vi "Vision Processing.vi"(4 "error in (no error)":errorcluster) -> ()   [LabVIEW 2013]
doc: "This VI runs in parallel to other tasks. It gets images from the camera, processes them for color or shape and use that information to affect robot behavior."
uses:
  Robot Global Data.vi
  <vilib>/Rock Robotics/WPI/Solenoid/Deprecated/WPI_SolenoidSetBool.vi
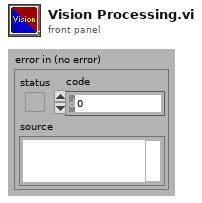
[diagram p1: front panel]
types:
  T1 = typedef "Image Type" = u32
  T2 = typedef "WPI_CameraDevRef.ctl" = cluster{"Camera Address":string, "CameraStatus":errorcluster, "Acquire Image Notifier":refnum<notifier>}
  T3 = typedef "IMAQ Image.ctl" = refnum<image>
  T4 = typedef "WPI_SolenoidDevRef.ctl" = cluster{"DevStatus":errorcluster, "Solenoid Module":T5, "Forward Solenoid Channel":T6, "Reverse Solenoid Channel":T6}
  T5 = typedef "FPGA_TypedefSolenoidModule.ctl" = enum16{"Solenoid Module 1", "Solenoid Module 2"}
  T6 = typedef "WPI_SolenoidChannel.ctl" = enum8{"Solenoid 1", "Solenoid 2", "Solenoid 3", "Solenoid 4", "Solenoid 5", "Solenoid 6", "Solenoid 7", "Solenoid 8", "Invalid"}
  T7 = typedef "WPI_CameraImageSize.ctl" = enum16{"640x480", "320x240", "160x120"}
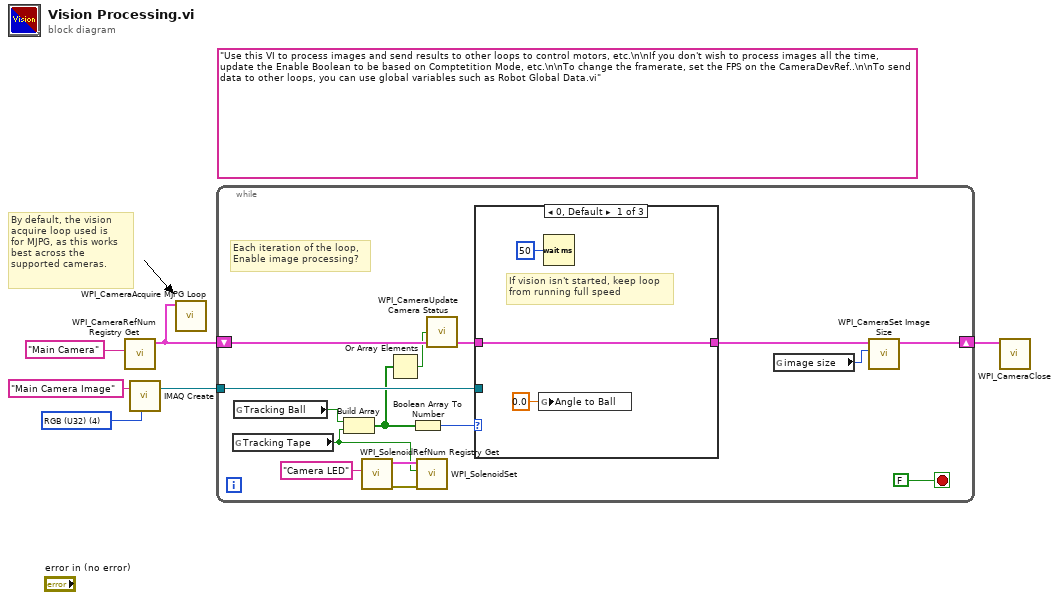
[diagram p0: block diagram]
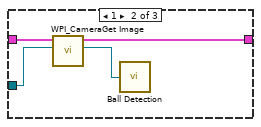
[diagram p2: hidden frame]
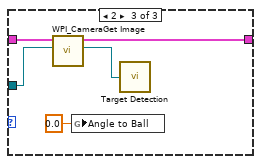
[diagram p3: hidden frame]
diagram:
  (unwired) "Use this VI to process images and send results to other loops to control motors, etc.\n\nIf you don't wish to process images all the time, update the Enable Boolean to be based on Comptetition Mode, etc.\n\nTo change the framerate, set the FPS on the CameraDevRef..\n\nTo send data to other loops, you can use global variables such as Robot Global Data.vi"
  w6 = T1 4 items=["Grayscale (U8)", "Grayscale (I16)", "Grayscale (SGL)", "Complex (CSG)", "RGB (U32)", "HSL (U32)", "RGB (U64)"] ("Image Type")
  # "By default, the vision\nacquire loop used is\nfor MJPG, as this works\nbest across the\nsupported cameras."
  n1 = call <vilib>:"WPI_CameraRefNum Registry Get.vi"("refnum name"="Main Camera") -> ("CameraDevRef"=w2:T2)  [unwired: 9 in, 1 out]
  n2 = call "IMAQ Create"("Image Name"="Main Camera Image", "Image Type"=w6) -> ("New Image"=w4:T3)  [unwired: 2 in, 2 out]
  n3 = call <vilib>:"WPI_CameraAcquire MJPG Loop.vi"("CameraDevRef"=w2) -> ()  [unwired: 11 in]
  n4 = while {
    shift-right: [w8] -> w1
    shift-left: w2 -> [w19]
    tunnel: w4 -> [w20]
    stop <- FALSE stop-if-true
    # "Each iteration of the loop,\nEnable image processing?"
    n5 = global read "Robot Global Data.vi" "Tracking Tape"() -> (w7:bool)
    n6 = global read "Robot Global Data.vi" "Tracking Ball"() -> (w17:bool)
    n7 = Build Array(w17, w7) -> (w15:bool[])
    n8 = call <vilib>:"WPI_SolenoidRefNum Registry Get.vi"("refnum name"="Camera LED") -> ("error out"=w12:errorcluster, "SolenoidDevRef"=w13:T4)  [unwired: 9 in]
    n9 = Or Array Elements(Boolean array=w15) -> (logical OR=w14:bool)
    n10 = Boolean Array To Number(Boolean array=w15) -> (number=w16:u32)
    n11 = call-poly <vilib>:"WPI_SolenoidSet.vi"("error in (no error)"=w12, "Value"=w7, "SolenoidDevRef"=w13) -> ()  [unwired: 7 in, 2 out]
    n12 = call <vilib>:"WPI_CameraUpdate Camera Status.vi"("CameraDevRef In"=w19, "Enable Vision"=w14) -> ("CameraDevRef Out"=w18:T2)  [unwired: 3 in]
    n13 = case shown="0, Default" w16 {
      tunnel: w20 -> [_ w28 w33]
      tunnel: [w24 w25 w29] -> w9
      tunnel: w18 -> [w24 w27 w32]
      frame 0, Default {
        # "If vision isn't started, keep loop\nfrom running full speed"
        n14 = global write "Robot Global Data.vi" "Angle to Ball"(0.0 ("Angle to Ball")) -> ()
        n15 = Wait (ms)(milliseconds to wait=u32 50) -> ()  [unwired: 1 out]
      }
      frame 1 {
        n16 = call <vilib>:"WPI_CameraGet Image.vi"("Image"=w28, "CameraDevRef"=w27) -> ("Image Out"=w26:T3, "CameraDevRef Out"=w25:T2)  [unwired: 1 in, 7 out]
        n17 = call "Ball Detection.vi"("Camera Image"=w26) -> ()
      }
      frame 2 {
        n18 = call <vilib>:"WPI_CameraGet Image.vi"("Image"=w33, "CameraDevRef"=w32) -> ("Image Out"=w31:T3, "CameraDevRef Out"=w29:T2)  [unwired: 1 in, 7 out]
        n19 = global write "Robot Global Data.vi" "Angle to Ball"(0.0 ("Angle to Ball")) -> ()
        n20 = call "Target Detection.vi"("Camera Image"=w31) -> ()
      }
    }
    n21 = global read "Robot Global Data.vi" "image size"() -> (w10:T7)
    n22 = call <vilib>:"WPI_CameraSet Image Size.vi"("Image Size"=w10, "CameraDevRef"=w9) -> ("CameraDevRef Out"=w8:T2)  [unwired: 1 in, 8 out]
  }
  n23 = call <vilib>:"WPI_CameraClose.vi"("CameraDevRef"=w1) -> ()  [unwired: 1 in, 10 out]
